vi "CRYAna Frequency.vi"(0 "Option In":bool[](array[boolean]), 1 "Abs/Rel":u16(ring) items=["Absolute", "Relative"], 3 "Stimulus Infor":cluster{"Fs":dbl, "Amplitude":dbl}={"Fs"=180.0, "Amplitude"=180.0}, 5 "Stimulus":dbl[](array[numeric]), 9 "Response":dbl[](array[numeric]), 11 "Option":cluster{"Averaging":u16, "Spectral Scaling":u16}, 12 "Freq":dbl[](array[numeric]), 13 "Time cluster":T3, 14 "EQ information":T2={"Stimulus EQ Curve"={"Name"="", "Curve"=[], "X data"=1, "Y data"=1, "Z data"=1, "X axis"=0, "Y axis"=1, "Z axis"=1, "X unit"="Hz", "Y unit"="", "Z unit"="deg.", "X dB ref"=1.0, "Y dB ref"=1.0, "Z dB ref"=1.0, "single val"=FALSE, "protected"=FALSE, "display X"=TRUE, "display Y"=TRUE, "display Z"=TRUE, "Test Info"="", "Step No."=0, "Plot Settings"={"Color"=0, "Interpolation"=0, "Point Style"=0, "Line Style"=0, "Point Color"=0, "Line Width"=0, "Bar Plot Style"=0, "Fill To"=0}, "AutoProtect"=FALSE}, "EQ"=FALSE, "EQ Rate"=0.0} {"EQ Rate" format="%.2f"; "Stimulus EQ Curve"."Z data" items=["dB", "Lin"]; "Stimulus EQ Curve"."X data" items=["dB", "Lin"]; "Stimulus EQ Curve"."Y data" items=["dB", "Lin"]; "Stimulus EQ Curve"."Z dB ref" format="%.1f"; "Stimulus EQ Curve"."Z axis" items=["Log", "Lin"]; "Stimulus EQ Curve"."X dB ref" format="%.1f"; "Stimulus EQ Curve"."X axis" items=["Log", "Lin"]; "Stimulus EQ Curve"."Y axis" items=["Log", "Lin"]; "Stimulus EQ Curve"."Y dB ref" format="%.1f"; "Stimulus EQ Curve"."Curve"."z" format="%.2f"; "Stimulus EQ Curve"."Curve"."y" format="%.2f"; "Stimulus EQ Curve"."Curve"."x" format="%.2f"}) -> (10 "Curve Out":cluster{cluster{"cycles":dbl, dbl, dbl}[]}[](array[cluster]))   [LabVIEW 2013]
uses:
  Typedef Control/CRYData Cluster.ctl
panel:
  out "XY Graph":cluster{dbl, dbl, "element":dbl}[](graph)
  out "Waveform Graph":dbl[](graph)
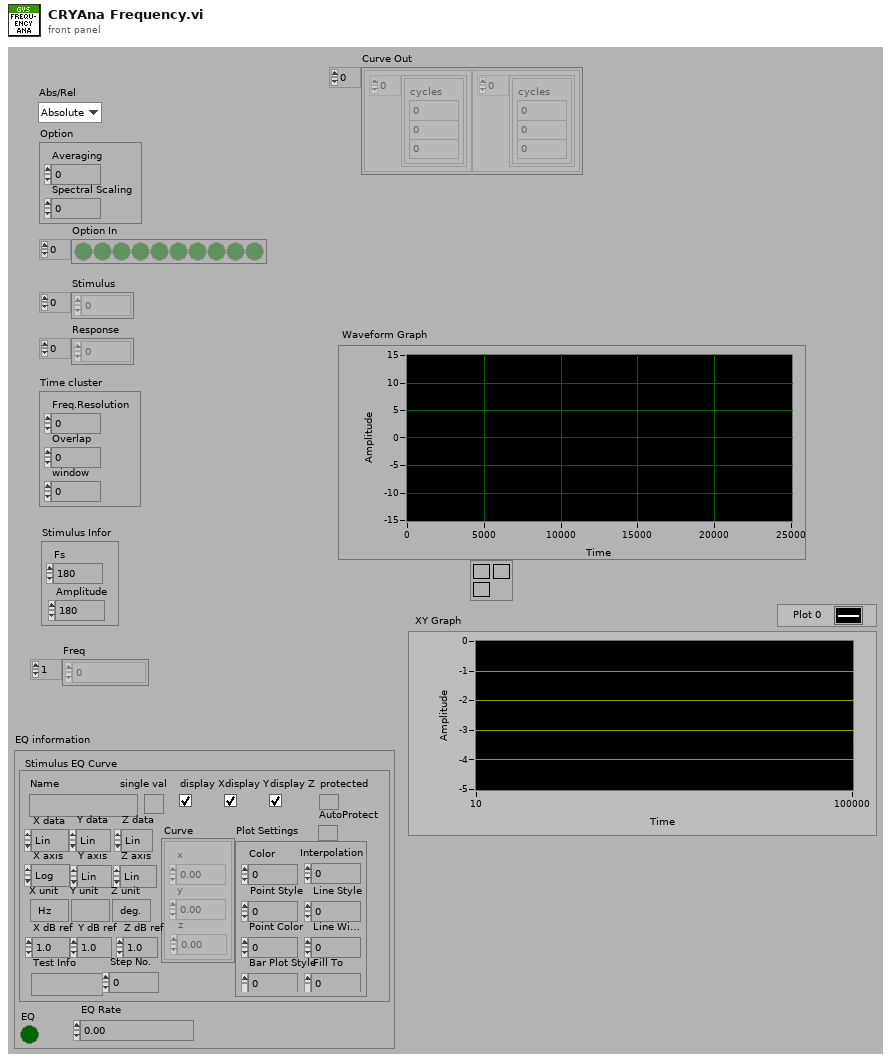
[diagram p1: front panel]
types:
  T1 = typedef "CRYData Cluster.ctl" = cluster{"Name":string, "Curve":cluster{"x":dbl, "y":dbl, "z":dbl}[], "X data":u16, "Y data":u16, "Z data":u16, "X axis":u16, "Y axis":u16, "Z axis":u16, "X unit":string, "Y unit":string, "Z unit":string, "X dB ref":dbl, "Y dB ref":dbl, "Z dB ref":dbl, "single val":bool, "protected":bool, "display X":bool, "display Y":bool, "display Z":bool, "Test Info":string, "Step No.":i32, "Plot Settings":cluster{"Color":u32, "Interpolation":u8, "Point Style":u8, "Line Style":u8, "Point Color":u32, "Line Width":u8, "Bar Plot Style":u8, "Fill To":i16}, "AutoProtect":bool}
  T2 = cluster{"Stimulus EQ Curve":T1, "EQ":bool, "EQ Rate":dbl}
  T3 = cluster{"Freq.Resolution":dbl, "Overlap":dbl, "window":u16}
  T4 = cluster{"Fs":dbl, "Freq.Resolution":dbl, "Overlap":dbl, "window":u16}
  T5 = cluster{cluster{"cycles":dbl, ext, "element":dbl}[]}[]
  T6 = cluster{cluster{"cycles":dbl, ext, "Phase In":dbl}[]}[]
  T7 = cluster{cluster{"cycles":dbl, ext, "Phase In":dbl}[]}
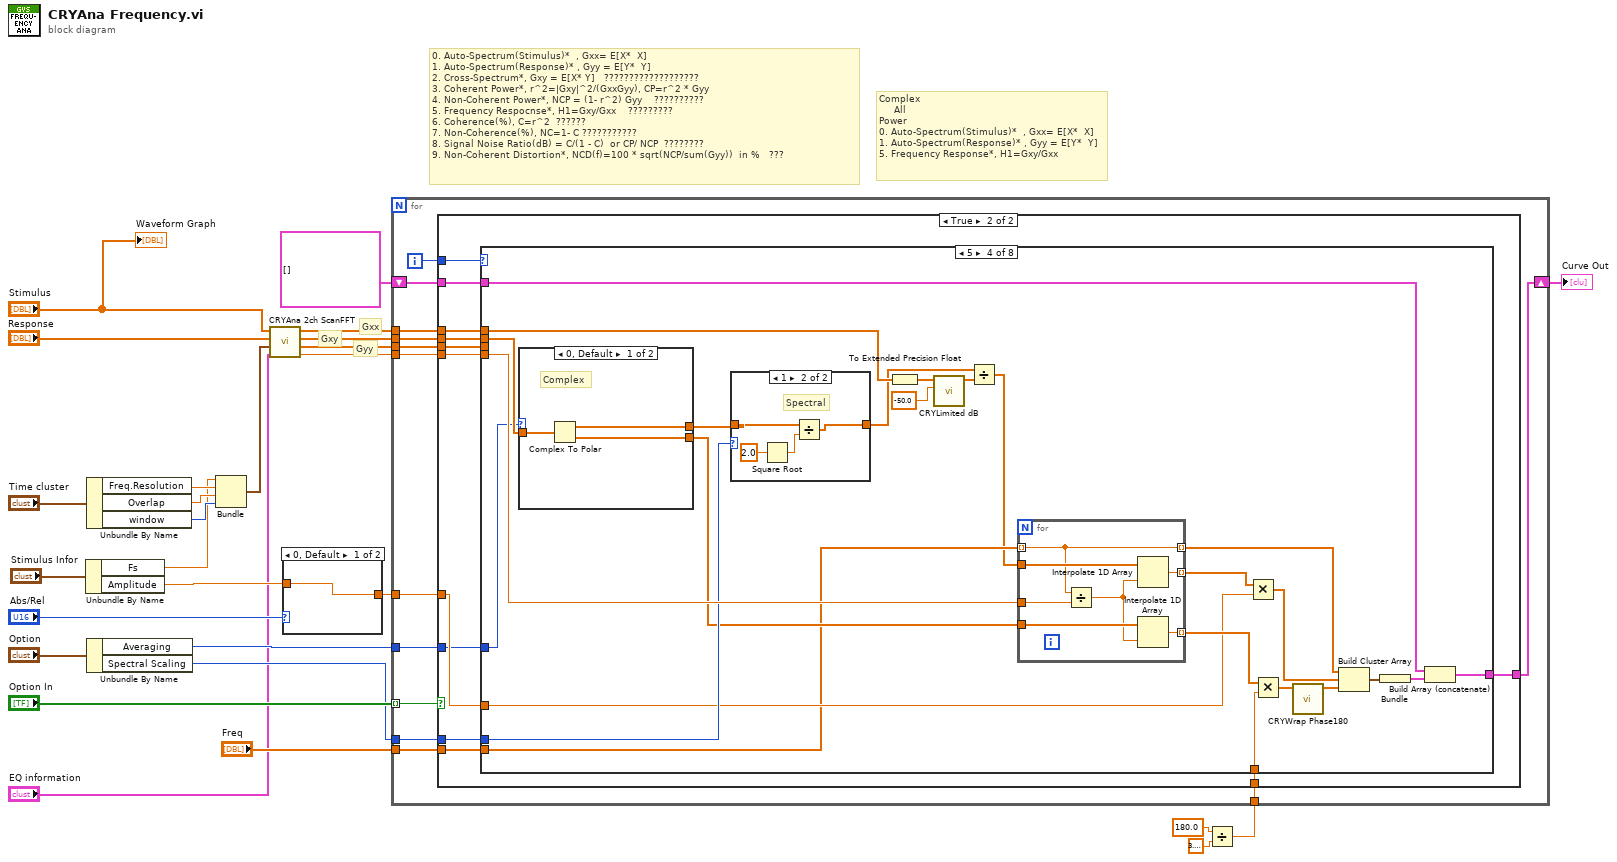
[diagram p0: block diagram]
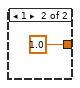
[diagram p2: hidden frame]
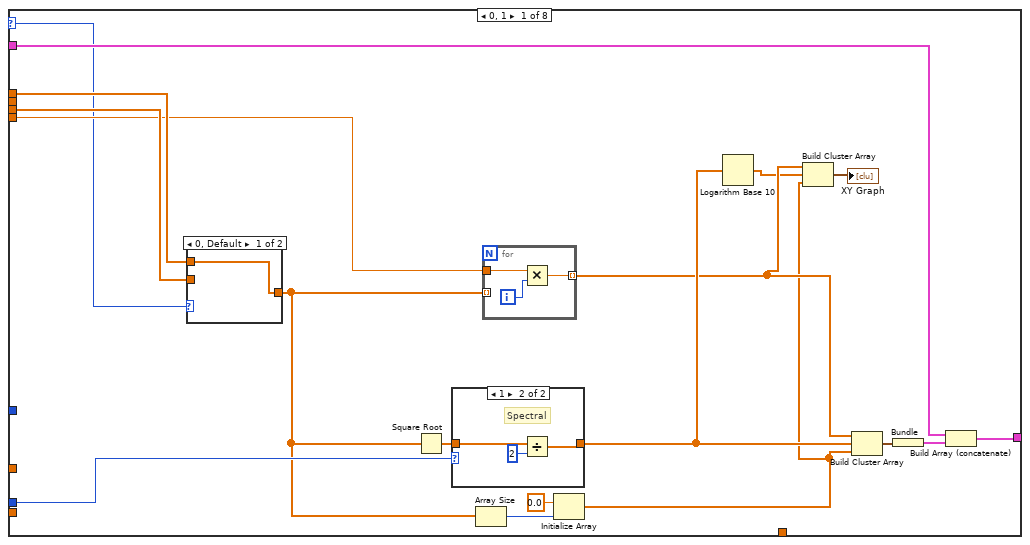
[diagram p4: hidden frame]
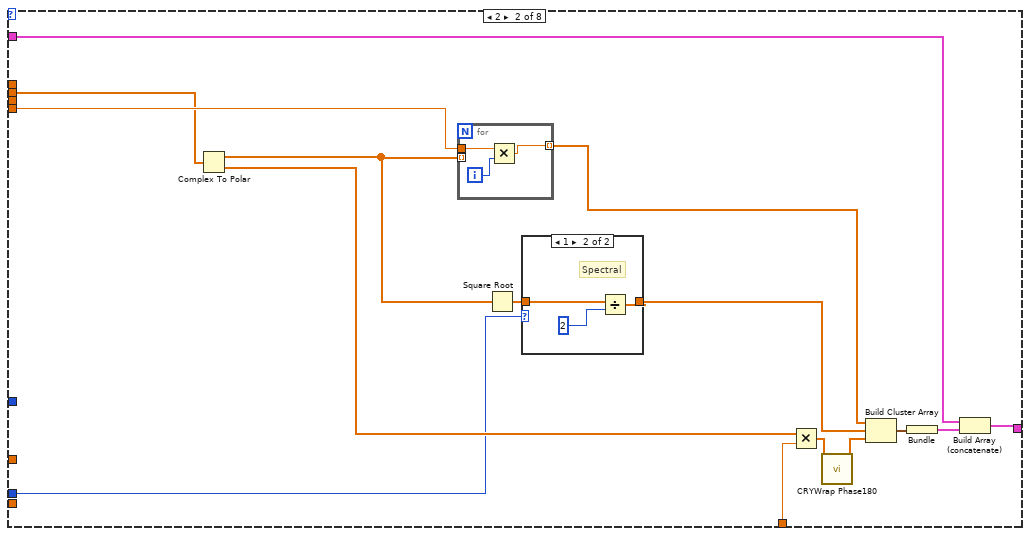
[diagram p7: hidden frame]
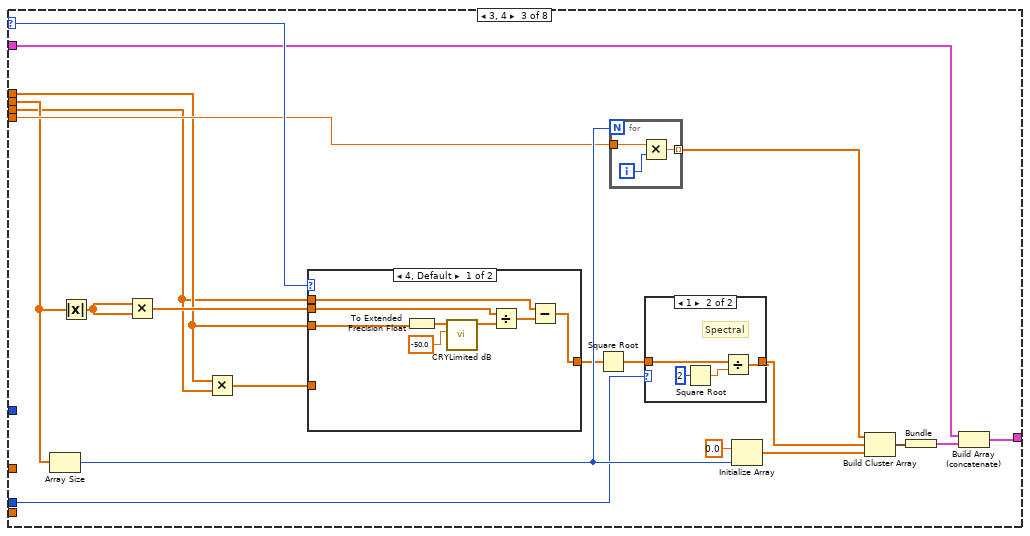
[diagram p9: hidden frame]
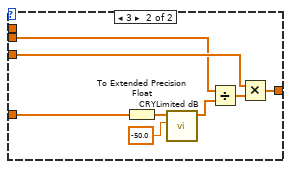
[diagram p11: hidden frame]
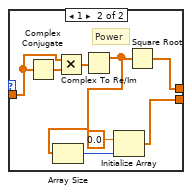
[diagram p12: hidden frame]
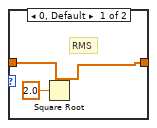
[diagram p13: hidden frame]
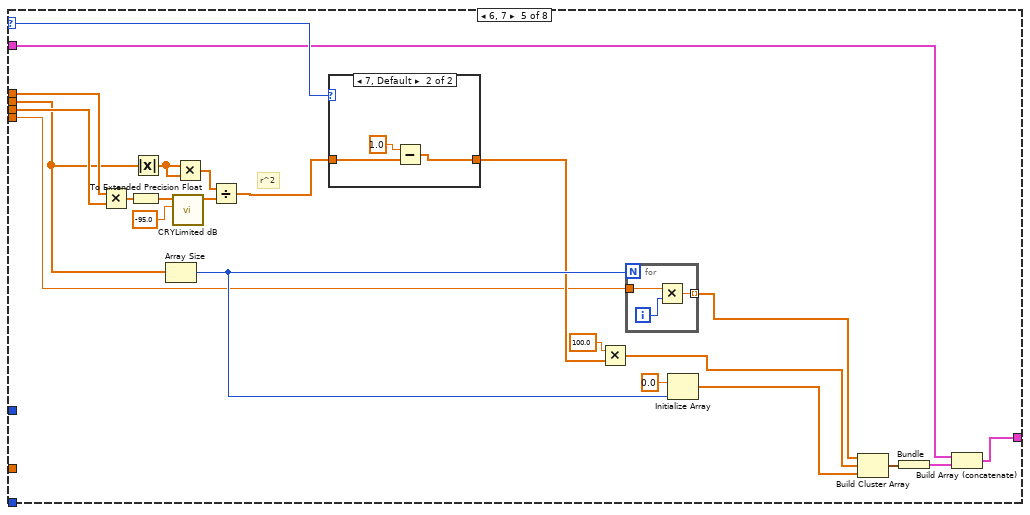
[diagram p14: hidden frame]
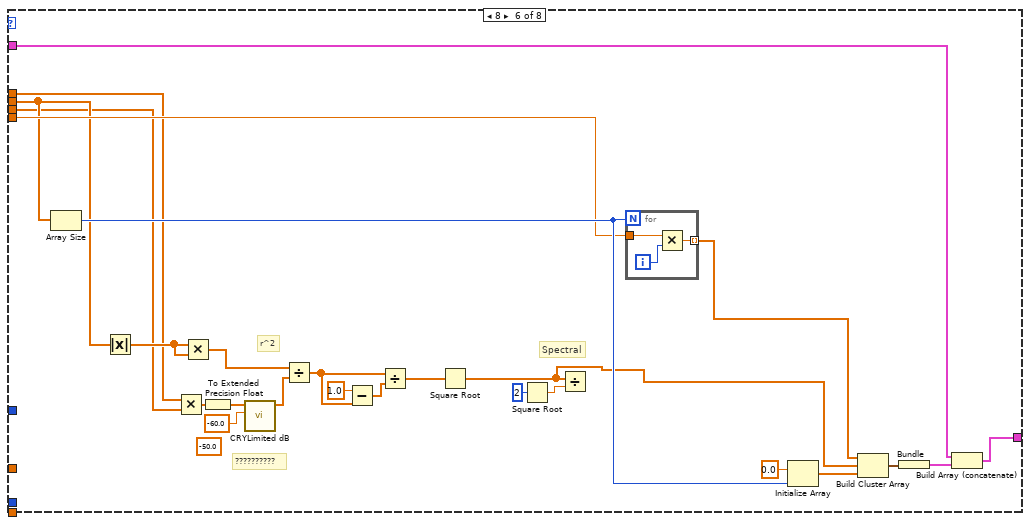
[diagram p16: hidden frame]
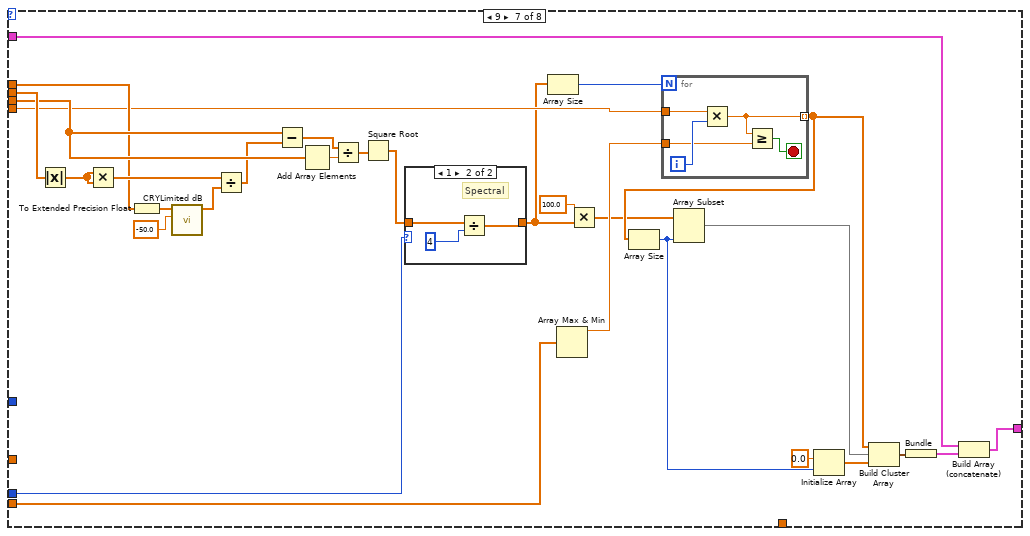
[diagram p17: hidden frame]
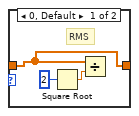
[diagram p18: hidden frame]
diagram:
  # "Complex\n     All\nPower\n0. Auto-Spectrum(Stimulus)*  , Gxx= E[X*  X]\n1. Auto-Spectrum(Response)* , Gyy = E[Y*  Y]\n5. Frequency Response*, H1=Gxy/Gxx"
  # "Gxy"
  # "0. Auto-Spectrum(Stimulus)*  , Gxx= E[X*  X]\n1. Auto-Spectrum(Response)* , Gyy = E[Y*  Y]\n2. Cross-Spectrum*, Gxy = E[X* Y]   ???????????????????\n3. Coherent Power*, r^2=|Gxy|^2/(GxxGyy), CP=r^2 * Gyy\n4. Non-Coherent Power*, NCP = (1- r^2) Gyy    ??????????\n5. Frequency Respocnse*, H1=Gxy/Gxx    ?????????\n6. Coherence(%), C=r^2  ??????\n7. Non-Coherence(%), NC=1- C ???????????\n8. Signal Noise Ratio(dB) = C/(1 - C)  or CP/ NCP  ????????\n9. Non-Coherent Distortion*, NCD(f)=100 * sqrt(NCP/sum(Gyy))  in %   ???"
  # "Gxx"
  # "Gyy"
  n1 = Unbundle By Name("Stimulus Infor") -> ("Fs"=w5:dbl, "Amplitude"=w4:dbl)
  n2 = Unbundle By Name("Time cluster") -> ("Freq.Resolution"=w17:dbl, "Overlap"=w16:dbl, "window"=w15:u16)
  n3 = Unbundle By Name("Option") -> ("Averaging"=w10:u16, "Spectral Scaling"=w14:u16)
  n4 = Bundle("Fs"=w5, "Freq.Resolution"=w17, "Overlap"=w16, "window"=w15) -> (w19:T4)  [unwired: 1 in]
  n5 = call "CRYAna 2ch ScanFFT.vi"("EQ information"="EQ information", "In Parameter"=w19, "Response[y(t)]"="Response", "Stimulus[x(t)]"="Stimulus") -> ("New dF(Hz)"=w20:dbl, "Gyy"=w11:dbl[], "Gxy"=w12:cdb[], "Gxx"=w13:dbl[])  [unwired: 4 in]
  n6 = case shown="0, Default" "Abs/Rel" {
    tunnel: [w28 1.0 ("Dynamic(dB)")] -> w7
    tunnel: w4 -> [w28 _]
    frame 0, Default {
    }
    frame 1 {
    }
  }
  n7 = Divide(x=180.0, y=3.141592653589793) -> (x/y=w21:dbl)
  n8 = for {
    tunnel: "Option In" -> [w41] mode=indexing
    shift-right: [w40] -> w25
    shift-left: cluster{cluster{dbl, dbl, dbl}[]}[] [] -> [w39]
    tunnel: w21 -> [w38]
    tunnel: w14 -> [w37]
    tunnel: w13 -> [w36]
    tunnel: w12 -> [w35]
    tunnel: w20 -> [w34]
    tunnel: w11 -> [w33]
    tunnel: w10 -> [w31]
    tunnel: w7 -> [w32]
    tunnel: "Freq" -> [w30]
    i -> [w42]
    n9 = case shown="True" w41 {
      tunnel: w42 -> [_ w55]
      tunnel: [w43 w54] -> w40
      tunnel: w39 -> [w43 w53]
      tunnel: w38 -> [_ w52]
      tunnel: w37 -> [_ w51]
      tunnel: w36 -> [_ w50]
      tunnel: w35 -> [_ w49]
      tunnel: w34 -> [_ w48]
      tunnel: w33 -> [_ w47]
      tunnel: w32 -> [_ w46]
      tunnel: w31 -> [_ w45]
      tunnel: w30 -> [_ w44]
      frame False {
      }
      frame True {
        n10 = case shown="5" w55 {
          selector: w55 -> [w66 _ w122 _ w217 _ _ _]
          tunnel: [w70 w95 w119 w170 w212 w246 w280 w297] -> w54
          tunnel: w53 -> [w71 w93 w117 w171 w213 w247 w279 w297]
          tunnel: w52 -> [_ w92 _ w169 _ _ _ _]
          tunnel: w51 -> [w65 w86 w113 w163 _ _ w275 _]
          tunnel: w50 -> [w69 _ w107 w160 w209 w233 w268 _]
          tunnel: w49 -> [_ w90 w109 w161 w204 w240 w277 _]
          tunnel: w48 -> [w67 w91 w114 w165 w206 w243 w263 _]
          tunnel: w47 -> [w68 _ w106 _ w208 w239 w269 _]
          tunnel: w46 -> [_ _ _ w157 _ _ _ _]
          tunnel: w45 -> [_ _ _ w155 _ _ _ _]
          tunnel: w44 -> [_ _ _ w154 _ _ w264 _]
          frame 0, 1 {
            n11 = case shown="0, Default" w66 {
              tunnel: w69 -> [w78 _]
              tunnel: w68 -> [_ w79]
              tunnel: [w78 w79] -> w63
              frame 0, Default {
              }
              frame 1 {
              }
            }
            n12 = Square Root(x=w63) -> (sqrt(x)=w64:dbl[])
            n13 = case shown="1" w65 {
              tunnel: w64 -> [w74 w76]
              tunnel: [w74 w75] -> w60
              frame 0, Default {
                # "RMS"
              }
              frame 1 {
                # "Spectral"
                n14 = Divide(x=w76, y=2) -> (x/y=w75:dbl[])
              }
            }
            n15 = Array Size(array=w63) -> (size(s)=w72:i32)
            n16 = for {
              tunnel: [w80] -> w59 mode=indexing
              tunnel: w67 -> [w81]
              tunnel: w63 -> [_] mode=indexing
              i -> [w82]
              n17 = Multiply(x=w81, y=w82) -> (x*y=w80:dbl)
            }
            n18 = Initialize Array(0.0 ("element"), w72) -> (w57:dbl[])
            n19 = Logarithm Base 10(1:w60) -> (0:w58:dbl[])
            n20 = Build Cluster Array(w59, w58, w57) -> (→"XY Graph":cluster{dbl, dbl, "element":dbl}[])
            n21 = Build Cluster Array(w59, w60, w57) -> (w61:cluster{dbl, dbl, "element":dbl}[])
            n22 = Bundle(w61) -> (w62:cluster{cluster{dbl, dbl, "element":dbl}[]})  [unwired: 1 in]
            n23 = Build Array (concatenate)(w71, w62) -> (w70:T5)
          }
          frame 2 {
            n24 = Complex To Polar(r * e^(i*theta)=w90) -> (r=w87:dbl[], theta=w89:dbl[])
            n25 = for {
              tunnel: w91 -> [w104]
              tunnel: [w102] -> w94 mode=indexing
              tunnel: w87 -> [_] mode=indexing
              i -> [w103]
              n26 = Multiply(x=w104, y=w103) -> (x*y=w102:dbl)
            }
            n27 = Square Root(x=w87) -> (sqrt(x)=w88:dbl[])
            n28 = case shown="1" w86 {
              tunnel: w88 -> [w98 w101]
              tunnel: [w98 w100] -> w85
              frame 0, Default {
                # "RMS"
              }
              frame 1 {
                # "Spectral"
                n29 = Divide(x=w101, y=2) -> (x/y=w100:dbl[])
              }
            }
            n30 = Multiply(x=w89, y=w92) -> (x*y=w84:dbl[])
            n31 = call "CRYWrap Phase180.vi"("Phase In"=w84) -> ("Phase Out"=w83:dbl[])  [unwired: 10 in]
            n32 = Build Cluster Array(w94, w85, w83) -> (w97:cluster{dbl, dbl, "Phase In":dbl}[])
            n33 = Bundle(w97) -> (w96:cluster{cluster{dbl, dbl, "Phase In":dbl}[]})  [unwired: 1 in]
            n34 = Build Array (concatenate)(w93, w96) -> (w95:T6)
          }
          frame 3, 4 {
            n35 = Array Size(array=w109) -> (size(s)=w123:i32)
            n36 = Absolute Value(x=w109) -> (abs(x)=w115:dbl[])
            n37 = Multiply(x=w115, y=w115) -> (x*y=w108:dbl[])
            n38 = Multiply(x=w107, y=w106) -> (x*y=w105:dbl[])
            n39 = case shown="4, Default" w122 {
              tunnel: w107 -> [w135 w145]
              tunnel: [w130 w144] -> w112
              tunnel: w108 -> [w133 w143]
              tunnel: w106 -> [w131 _]
              tunnel: w105 -> [_ w139]
              frame 4, Default {
                n40 = To Extended Precision Float(1:w135) -> (0:w136:ext[])
                n41 = call "CRYLimited dB.vi"("Dynamic(dB)"=-50.0, "Power spectrum"=w136) -> ("Limited spectrum"=w134:ext[])  [unwired: 9 in]
                n42 = Divide(x=w133, y=w134) -> (x/y=w132:ext[])
                n43 = Subtract(x=w131, y=w132) -> (x-y=w130:ext[])
              }
              frame 3 {
                n44 = To Extended Precision Float(1:w139) -> (0:w141:ext[])
                n45 = call "CRYLimited dB.vi"("Dynamic(dB)"=-50.0, "Power spectrum"=w141) -> ("Limited spectrum"=w138:ext[])  [unwired: 9 in]
                n46 = Divide(x=w143, y=w138) -> (x/y=w142:ext[])
                n47 = Multiply(x=w145, y=w142) -> (x*y=w144:ext[])
              }
            }
            n48 = Square Root(x=w112) -> (sqrt(x)=w110:ext[])
            n49 = for {
              N: w123 -> [_]
              tunnel: w114 -> [w148]
              tunnel: [w146] -> w118 mode=indexing
              i -> [w147]
              n50 = Multiply(x=w148, y=w147) -> (x*y=w146:dbl)
            }
            n51 = case shown="1" w113 {
              tunnel: w110 -> [w125 w129]
              tunnel: [w125 w128] -> w111
              frame 0, Default {
                # "RMS"
              }
              frame 1 {
                # "Spectral"
                n52 = Square Root(x=2) -> (sqrt(x)=w126:dbl)
                n53 = Divide(x=w129, y=w126) -> (x/y=w128:ext[])
              }
            }
            n54 = Initialize Array(0.0 ("element"), w123) -> (w116:dbl[])
            n55 = Build Cluster Array(w118, w111, w116) -> (w121:cluster{dbl, ext, "element":dbl}[])
            n56 = Bundle(w121) -> (w120:cluster{cluster{dbl, ext, "element":dbl}[]})  [unwired: 1 in]
            n57 = Build Array (concatenate)(w117, w120) -> (w119:T5)
          }
          frame 5 {
            n58 = case shown="0, Default" w155 {
              tunnel: [w175 w182] -> w162
              tunnel: w161 -> [w176 w179]
              tunnel: [w174 w178] -> w152
              frame 0, Default {
                # "Complex"
                n59 = Complex To Polar(r * e^(i*theta)=w176) -> (r=w174:dbl[], theta=w175:dbl[])
              }
              frame 1 {
                # "Power"
                n60 = Complex Conjugate(1:w179) -> (0:w181:cdb[])
                n61 = Multiply(x=w179, y=w181) -> (x*y=w180:cdb[])
                n62 = Complex To Re/Im(x + iy=w180) -> (x=w177:dbl[])  [unwired: 1 out]
                n63 = Array Size(array=w177) -> (size(s)=w183:i32)
                n64 = Initialize Array(0.0 ("element"), w183) -> (w182:dbl[])
                n65 = Square Root(x=w177) -> (sqrt(x)=w178:dbl[])
              }
            }
            n66 = case shown="1" w163 {
              tunnel: w152 -> [w185 w190]
              tunnel: [w185 w189] -> w153
              frame 0, Default {
                # "RMS"
                n67 = Square Root(x=2.0) -> ()  [unwired: 1 out]
              }
              frame 1 {
                # "Spectral"
                n68 = Square Root(x=2.0) -> (sqrt(x)=w187:dbl)
                n69 = Divide(x=w190, y=w187) -> (x/y=w189:dbl[])
              }
            }
            n70 = To Extended Precision Float(1:w160) -> (0:w167:ext[])
            n71 = call "CRYLimited dB.vi"("Dynamic(dB)"=-50.0, "Power spectrum"=w167) -> ("Limited spectrum"=w166:ext[])  [unwired: 9 in]
            n72 = Divide(x=w153, y=w166) -> (x/y=w151:ext[])
            n73 = for {
              tunnel: w154 -> [w193] mode=indexing
              tunnel: w151 -> [w197]
              tunnel: [w196] -> w158 mode=indexing
              tunnel: w165 -> [w192]
              tunnel: [w193] -> w159 mode=indexing
              tunnel: w162 -> [w195]
              tunnel: [w194] -> w164 mode=indexing
              n74 = Divide(x=w193, y=w192) -> (x/y=w191:dbl)
              n75 = Interpolate 1D Array(1:w191, 2:w197) -> (0:w196:ext)
              n76 = Interpolate 1D Array(1:w191, 2:w195) -> (0:w194:dbl)
            }
            n77 = Multiply(x=w158, y=w157) -> (x*y=w156:ext[])
            n78 = Multiply(x=w164, y=w169) -> (x*y=w150:dbl[])
            n79 = call "CRYWrap Phase180.vi"("Phase In"=w150) -> ("Phase Out"=w149:dbl[])  [unwired: 10 in]
            n80 = Build Cluster Array(w159, w156, w149) -> (w173:cluster{"cycles":dbl, ext, "Phase In":dbl}[])
            n81 = Bundle(w173) -> (w172:T7)  [unwired: 1 in]
            n82 = Build Array (concatenate)(w171, w172) -> (w170:T6)
          }
          frame 6, 7 {
            # "r^2"
            n83 = Multiply(x=w209, y=w208) -> (x*y=w199:dbl[])
            n84 = To Extended Precision Float(1:w199) -> (0:w200:ext[])
            n85 = Absolute Value(x=w204) -> (abs(x)=w203:dbl[])
            n86 = Array Size(array=w204) -> (size(s)=w219:i32)
            n87 = call "CRYLimited dB.vi"("Dynamic(dB)"=-95.0, "Power spectrum"=w200) -> ("Limited spectrum"=w198:ext[])  [unwired: 9 in]
            n88 = Multiply(x=w203, y=w203) -> (x*y=w210:dbl[])
            n89 = Divide(x=w210, y=w198) -> (x/y=w202:ext[])
            n90 = case shown="7, Default" w217 {
              tunnel: w202 -> [w221 w223]
              tunnel: [w221 w222] -> w207
              frame 6 {
              }
              frame 7, Default {
                n91 = Subtract(x=1.0, y=w223) -> (x-y=w222:ext[])
              }
            }
            n92 = Multiply(x=100.0 ("element"), y=w207) -> (x*y=w205:ext[])
            n93 = for {
              N: w219 -> [_]
              tunnel: w206 -> [w227]
              tunnel: [w225] -> w214 mode=indexing
              i -> [w226]
              n94 = Multiply(x=w227, y=w226) -> (x*y=w225:dbl)
            }
            n95 = Initialize Array(0.0 ("element"), w219) -> (w211:dbl[])
            n96 = Build Cluster Array(w214, w205, w211) -> (w216:cluster{dbl, ext, "element":dbl}[])
            n97 = Bundle(w216) -> (w215:cluster{cluster{dbl, ext, "element":dbl}[]})  [unwired: 1 in]
            n98 = Build Array (concatenate)(w213, w215) -> (w212:T5)
          }
          frame 8 {
            (unwired) -50.0 ("Dynamic(dB)")
            # "??????????"
            # "Spectral"
            # "r^2"
            n99 = Array Size(array=w240) -> (size(s)=w251:i32)
            n100 = Absolute Value(x=w240) -> (abs(x)=w241:dbl[])
            n101 = Multiply(x=w233, y=w239) -> (x*y=w235:dbl[])
            n102 = Multiply(x=w241, y=w241) -> (x*y=w242:dbl[])
            n103 = To Extended Precision Float(1:w235) -> (0:w236:ext[])
            n104 = call "CRYLimited dB.vi"("Dynamic(dB)"=-60.0, "Power spectrum"=w236) -> ("Limited spectrum"=w234:ext[])  [unwired: 9 in]
            n105 = Divide(x=w242, y=w234) -> (x/y=w238:ext[])
            n106 = Subtract(x=1.0, y=w238) -> (x-y=w232:ext[])
            n107 = Divide(x=w238, y=w232) -> (x/y=w231:ext[])
            n108 = Square Root(x=w231) -> (sqrt(x)=w228:ext[])
            n109 = Square Root(x=2) -> (sqrt(x)=w229:dbl)
            n110 = Divide(x=w228, y=w229) -> ()  [unwired: 1 out]
            n111 = for {
              N: w251 -> [_]
              tunnel: w243 -> [w255]
              tunnel: [w253] -> w248 mode=indexing
              i -> [w254]
              n112 = Multiply(x=w255, y=w254) -> (x*y=w253:dbl)
            }
            n113 = Initialize Array(0.0 ("element"), w251) -> (w244:dbl[])
            n114 = Build Cluster Array(w248, w228, w244) -> (w250:cluster{dbl, ext, "element":dbl}[])
            n115 = Bundle(w250) -> (w249:cluster{cluster{dbl, ext, "element":dbl}[]})  [unwired: 1 in]
            n116 = Build Array (concatenate)(w247, w249) -> (w246:T5)
          }
          frame 9 {
            n117 = Absolute Value(x=w277) -> (abs(x)=w276:dbl[])
            n118 = Multiply(x=w276, y=w276) -> (x*y=w270:dbl[])
            n119 = To Extended Precision Float(1:w268) -> (0:w272:ext[])
            n120 = call "CRYLimited dB.vi"("Dynamic(dB)"=-50.0, "Power spectrum"=w272) -> ("Limited spectrum"=w271:ext[])  [unwired: 9 in]
            n121 = Divide(x=w270, y=w271) -> (x/y=w267:ext[])
            n122 = Subtract(x=w269, y=w267) -> (x-y=w266:ext[])
            n123 = Add Array Elements(numeric array=w269) -> (sum=w284:dbl)
            n124 = Divide(x=w266, y=w284) -> (x/y=w274:ext[])
            n125 = Square Root(x=w274) -> (sqrt(x)=w265:ext[])
            n126 = case shown="1" w275 {
              tunnel: w265 -> [w291 w296]
              tunnel: [w291 w294] -> w257
              frame 0, Default {
                # "RMS"
                n127 = Square Root(x=2) -> (sqrt(x)=w293:dbl)
                n128 = Divide(x=w291, y=w293) -> ()  [unwired: 1 out]
              }
              frame 1 {
                # "Spectral"
                n129 = Divide(x=w296, y=4) -> (x/y=w294:ext[])
              }
            }
            n130 = Array Size(array=w257) -> (size(s)=w256:i32)
            n131 = Array Max & Min(array=w264) -> (max value=w262:dbl)  [unwired: 3 out]
            n132 = Multiply(x=100.0 ("element"), y=w257) -> (x*y=w260:ext[])
            n133 = for {
              N: w256 -> [_]
              tunnel: w263 -> [w290]
              tunnel: w262 -> [w287]
              tunnel: [w288] -> w261 mode=indexing
              i -> [w289]
              stop <- w286 stop-if-true
              n134 = Multiply(x=w290, y=w289) -> (x*y=w288:dbl)
              n135 = Greater Or Equal?(x=w288, y=w287) -> (x >= y?=w286:bool)
            }
            n136 = Array Size(array=w261) -> (size(s)=w258:i32)
            n137 = Array Subset(array=w260, length=w258) -> (w259:ext[])  [unwired: 1 in]
            n138 = Initialize Array(0.0 ("element"), w258) -> (w278:dbl[])
            n139 = Build Cluster Array(w261, w259, w278) -> (w282:cluster{dbl, ext, "element":dbl}[])
            n140 = Bundle(w282) -> (w281:cluster{cluster{dbl, ext, "element":dbl}[]})  [unwired: 1 in]
            n141 = Build Array (concatenate)(w279, w281) -> (w280:T5)
          }
          frame Default {
          }
        }
      }
    }
  }
  "Curve Out" <- w25
  "Waveform Graph" <- "Stimulus"
